vi "Create user events.vi"(8 "error in (no error)":errorcluster) -> (0 "error out":errorcluster, 3 "event cluster":T1)   [LabVIEW 2020, in "FCR100.lvlib"]
uses:
  FCR100.lvlib
  Device state -- enum.ctl
  Wake HL data -- cluster.ctl
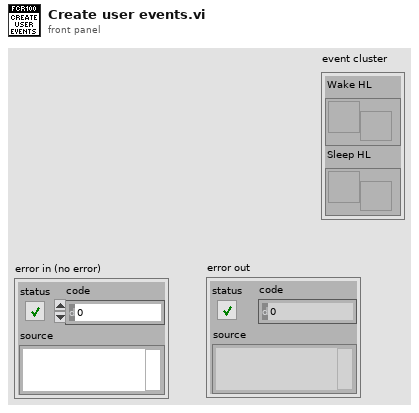
[diagram p1: front panel]
types:
  T1 = cluster{"Wake HL":refnum<user-event>, "Sleep HL":refnum<user-event>}
  T2 = typedef "FCR100.lvlib/Wake HL data -- cluster.ctl" = cluster{"Timeout":i32, "Instrument Channel":string, "Address":u8, "Current state":T3, "Desired state":T3, "Module ID":i32}
  T3 = typedef "FCR100.lvlib/Device state -- enum.ctl" = enum16{"Not referenced", "Configuration", "Disable", "Ready", "Homing", "Motion"}
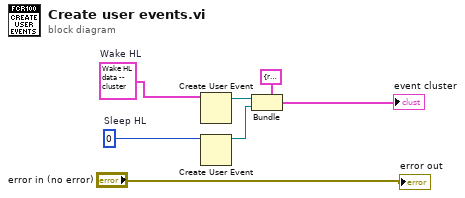
[diagram p0: block diagram]
diagram:
  w3 = u8 0  # Sleep HL
  w5 = T2 {"Timeout"=0, "Instrument Channel"="", "Address"=0, "Current state"=enum."Configuration", "Desired state"=enum."Configuration", "Module ID"=0}  # Wake HL
  n1 = Create User Event(user event datatype=w5) -> (user event=w6:refnum<user-event>)  [unwired: 1 in, 1 out]
  n2 = Create User Event(user event datatype=w3) -> (user event=w7:refnum<user-event>)  [unwired: 1 in, 1 out]
  n3 = Bundle(cluster=T1 {"Wake HL"=refnum, "Sleep HL"=refnum}, "Wake HL"=w6, "Sleep HL"=w7) -> (→"event cluster":T1)
  "error out" <- "error in (no error)"
